vi "Extract Single File.vi"(5 "Overwrite":bool, 7 "Return as String (F: Extract to File)":bool, 8 "error in (no error)":errorcluster, 9 "name or relative path (\"\": use output file name)":string, 10 "File output Path (extract to temp file)":path, 11 "Zip File Path":path) -> (0 "error out":errorcluster, 1 "String":string, 2 "Extracted File Path":path, 3 "dup Zip File Path":path)   [LabVIEW 2019, in "Command-Line Zip.lvlib"]
uses:
  Command-Line Zip.lvlib
  <userlib>/_OpenG.lib/file/file.llb/Valid Path - Traditional__ogtk.vi
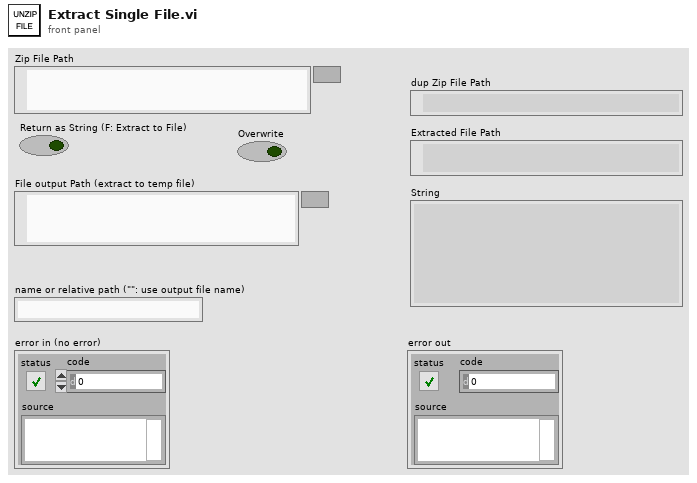
[diagram p1: front panel]
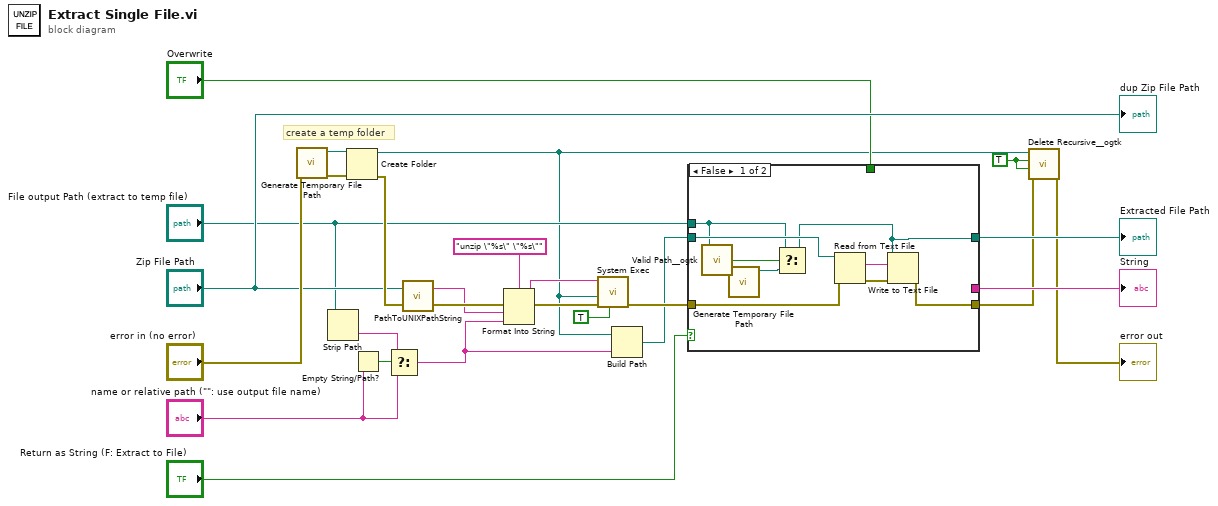
[diagram p0: block diagram]
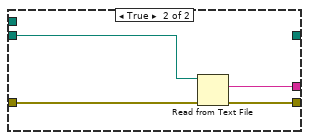
[diagram p2: hidden frame]
diagram:
  w4 = TRUE ("Recursive? (FALSE)")
  # "create a temp folder"
  n1 = call <vilib>:"Generate Temporary File Path.vi"("error in (no error)"="error in (no error)") -> ("error out"=w18:errorcluster, "Unique Temporary File Path"=w19:path)  [unwired: 9 in]
  n2 = Strip Path(path="File output Path (extract to temp file)") -> (name=w8:string)  [unwired: 1 out]
  n3 = Create Folder(path (use dialog)=w19, error in=w18) -> (created path=w1:path, error out=w20:errorcluster)  [unwired: 1 in, 1 out]
  n4 = Empty String/Path?(string/path="name or relative path (\"\": use output file name)") -> (empty?=w9:bool)
  n5 = Select(t=w8, s=w9, f="name or relative path (\"\": use output file name)") -> (s? t:f=w6:string)
  n6 = call <vilib>:"PathToUNIXPathString.vi"("error in (no error)"=w20, "LV Path"="Zip File Path") -> ("error out"=w17:errorcluster, "UNIX Path"=w16:string)
  n7 = Format Into String(format string="unzip \"%s\" \"%s\"" ("command line"), error in=w17, w16, w6) -> (resulting string=w13:string, error out=w14:errorcluster)  [unwired: 1 in]
  n8 = call <vilib>:"System Exec.vi"("run minimized? (F)"=TRUE, "error in (no error)"=w14, "working directory"=w1, "command line"=w13) -> ("error out"=w22:errorcluster)  [unwired: 4 in, 3 out]
  n9 = Build Path(base path=w1, name or relative path=w6) -> (appended path=w21:path)
  n10 = case shown="False" "Return as String (F: Extract to File)" {
    tunnel: w21 -> [w30 w38]
    tunnel: "File output Path (extract to temp file)" -> [w27 _]
    tunnel: w22 -> [w34 w39]
    tunnel: [w35 w37] -> w2
    tunnel: [_ w36] -> w24
    tunnel: [w28 _] -> w26
    tunnel: "Overwrite" -> [_ _]
    frame False {
      n11 = call-poly <userlib>:"Valid Path__ogtk.vi"("path"=w27) -> ("valid"=w31:bool)
      n12 = call <vilib>:"Generate Temporary File Path.vi"() -> ("Unique Temporary File Path"=w29:path)  [unwired: 10 in, 1 out]
      n13 = Select(t=w27, s=w31, f=w29) -> (s? t:f=w28:path)
      n14 = Read from Text File(file (use dialog)=w30, error in=w34) -> (text=w32:string, error out=w33:errorcluster)  [unwired: 2 in, 2 out]
      n15 = Write to Text File(file (use dialog)=w28, text=w32, error in=w33) -> (error out=w35:errorcluster)  [unwired: 1 in, 2 out]
    }
    frame True {
      n16 = Read from Text File(file (use dialog)=w38, error in=w39) -> (text=w36:string, error out=w37:errorcluster)  [unwired: 2 in, 2 out]
    }
  }
  "Extracted File Path" <- w26
  "String" <- w24
  n17 = call <userlib>:"Delete Recursive__ogtk.vi"("error in (no error)"=w2, "Ignore Read-Only? (FALSE)"=w4, "Recursive? (FALSE)"=w4, "Path"=w1) -> ("error out"=→"error out":errorcluster)  [unwired: 6 in, 1 out]
  "dup Zip File Path" <- "Zip File Path"
